vi "Recondense_mercury.vi"(5 "Recondense-Monitor in":T1 {"He3-Pot Heater %" format="%#_4g"; "He3-Pot Setpoint" format="%#_4g"; "Sorb Heater %" format="%#_4g"; "Sorb Setpoint" format="%#_4g"; "He3 Temp2" format="%#_4g"; "He3 Temp 1" format="%#_4g"; "1K Temp" format="%#_4g"; "Sorb Temp" format="%#_4g"}, 6 "TempErrorsIn":T7, 7 "Mercury Reference In H3 Temp2":T3, 8 "Mercury Reference In H3 Temp1":T3, 9 "Mercury Reference In 1K":T3, 10 "Mercury Reference In Sorb":T3) -> (0 "TempErrorsOut":T6, 2 "Mercury Reference out":T2, 3 "Recondense-Monitor out":T1 {"He3-Pot Heater %" format="%#_4g"; "He3-Pot Setpoint" format="%#_4g"; "Sorb Heater %" format="%#_4g"; "Sorb Setpoint" format="%#_4g"; "He3 Temp2" format="%#_4g"; "He3 Temp 1" format="%#_4g"; "1K Temp" format="%#_4g"; "Sorb Temp" format="%#_4g"})   [LabVIEW 2019]
uses:
  Equipment/Mercury iXX/Public/Controls/Mercury Reference.ctl
  Equipment/Mercury iXX/Public/Controls/Comms Transport Layer.ctl
  Equipment/Mercury iXX/Private/Controls/Query Dynamic Reference.ctl
  Monitor Communication/Brosowski/TempErrors_in.ctl
  Monitor Communication/Brosowski/TempErrors.ctl
  Monitor Communication/Brosowski/Mercury_Reference_out.ctl
  Monitor Communication/Brosowski/BorowskiMonitor.ctl
  Global/Global Variables/Data_Display_global.vi
  Equipment/Mercury iXX/Public/Libraries/Temperature.lvlib
  Equipment/Mercury iXX/Public/Libraries/Control Loop.lvlib
  Equipment/Mercury iXX/Mercury iXX.lvlib
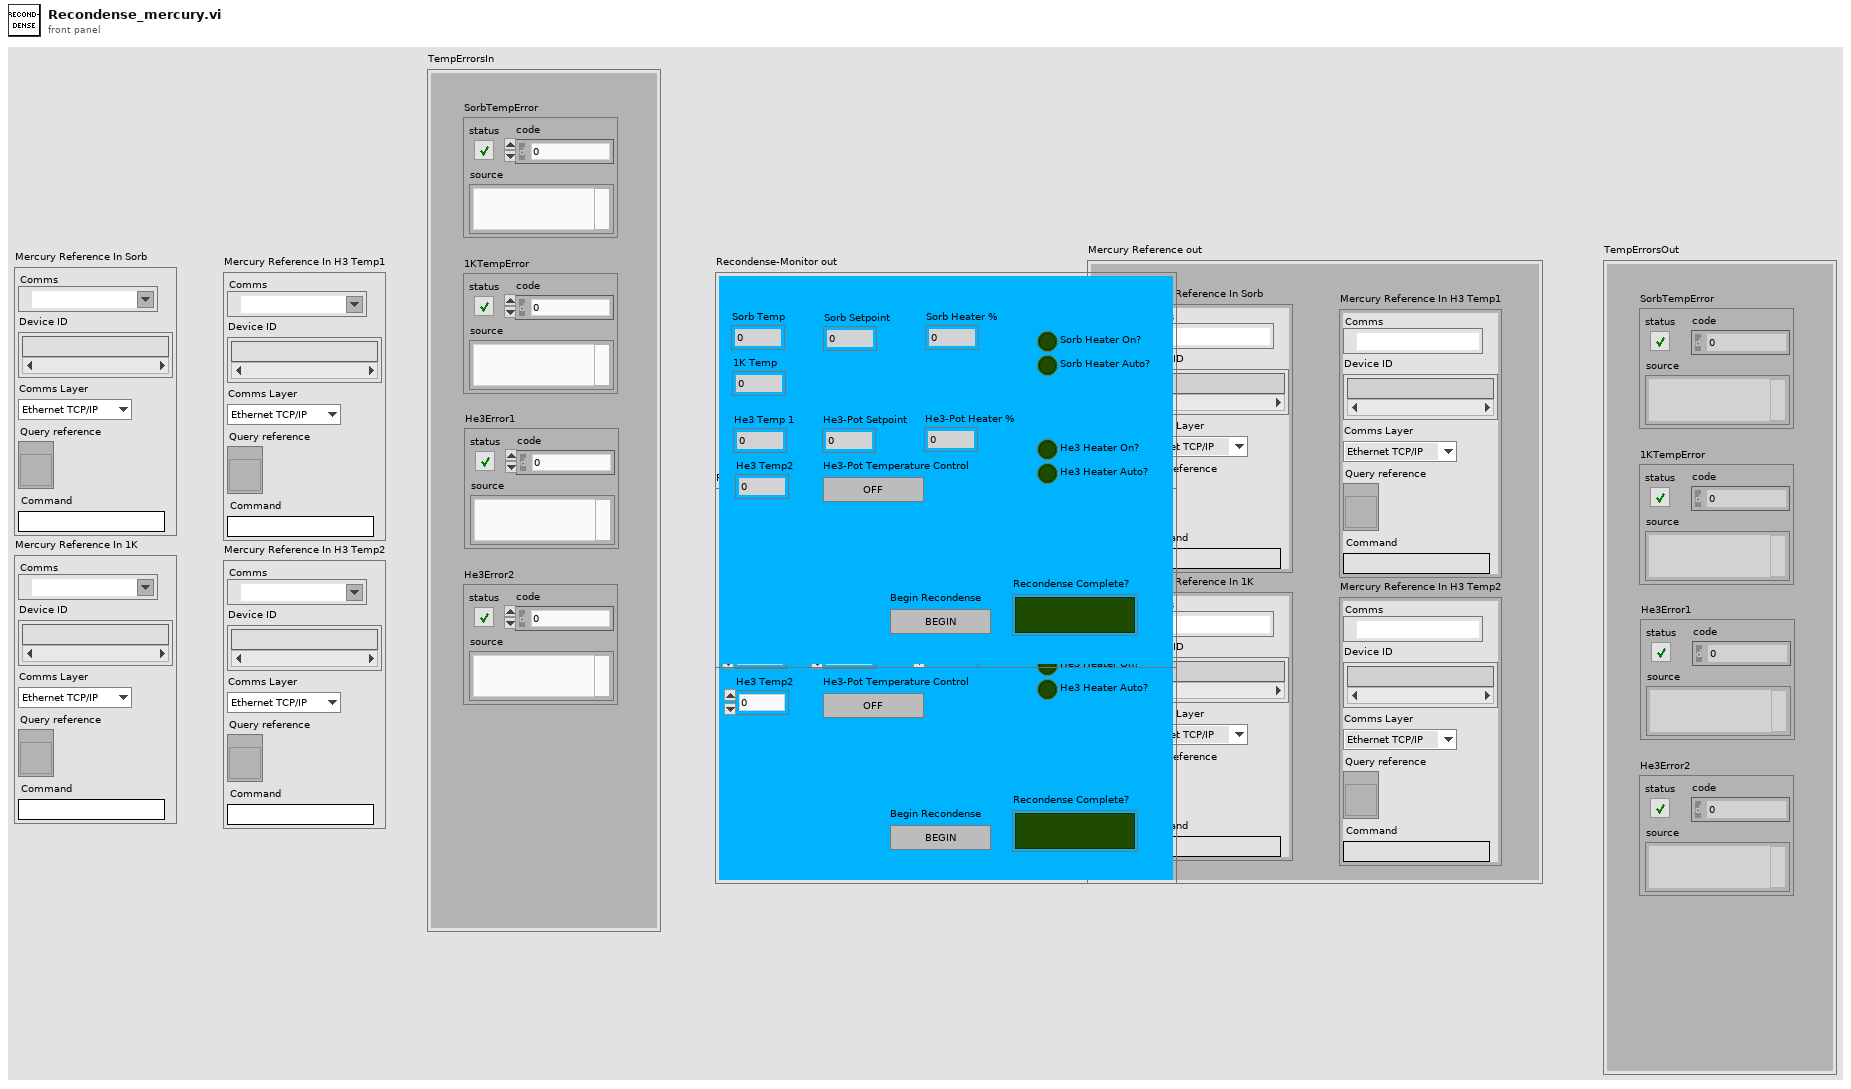
[diagram p1: front panel]
types:
  T1 = typedef "BorowskiMonitor.ctl" = cluster{"Sorb Temp":dbl, "1K Temp":dbl, "He3 Temp 1":dbl, "He3 Temp2":dbl, "Recondense Complete?":bool, "Sorb Heater Auto?":bool, "Sorb Heater On?":bool, "Sorb Setpoint":dbl, "Sorb Heater %":dbl, "Begin Recondense":bool, "He3-Pot Setpoint":dbl, "He3-Pot Heater %":dbl, "He3 Heater Auto?":bool, "He3 Heater On?":bool, "He3-Pot Temperature Control":bool}
  T2 = typedef "Mercury_Reference_out.ctl" = cluster{"Mercury Reference In Sorb":T3, "Mercury Reference In 1K":T3, "Mercury Reference In H3 Temp1":T3, "Mercury Reference In H3 Temp2":T3}
  T3 = typedef "Mercury iXX.lvlib/Mercury Reference.ctl" = cluster{"Comms":refnum<visa-resource-name>, "Device ID":string[], "Comms Layer":T4, "Command":string, "Query reference":T5}
  T4 = typedef "Mercury iXX.lvlib/Comms Transport Layer.ctl" = enum16{"Ethernet TCP/IP", "USB", "ISOBus - RS-232", "GPIB"}
  T5 = typedef "Mercury iXX.lvlib/Query Dynamic Reference.ctl" = refnum<vi>
  T6 = typedef "TempErrors.ctl" = cluster{"SorbTempError":errorcluster, "1KTempError":errorcluster, "He3Error1":errorcluster, "He3Error2":errorcluster}
  T7 = typedef "TempErrors_in.ctl" = cluster{"SorbTempError":errorcluster, "1KTempError":errorcluster, "He3Error1":errorcluster, "He3Error2":errorcluster}
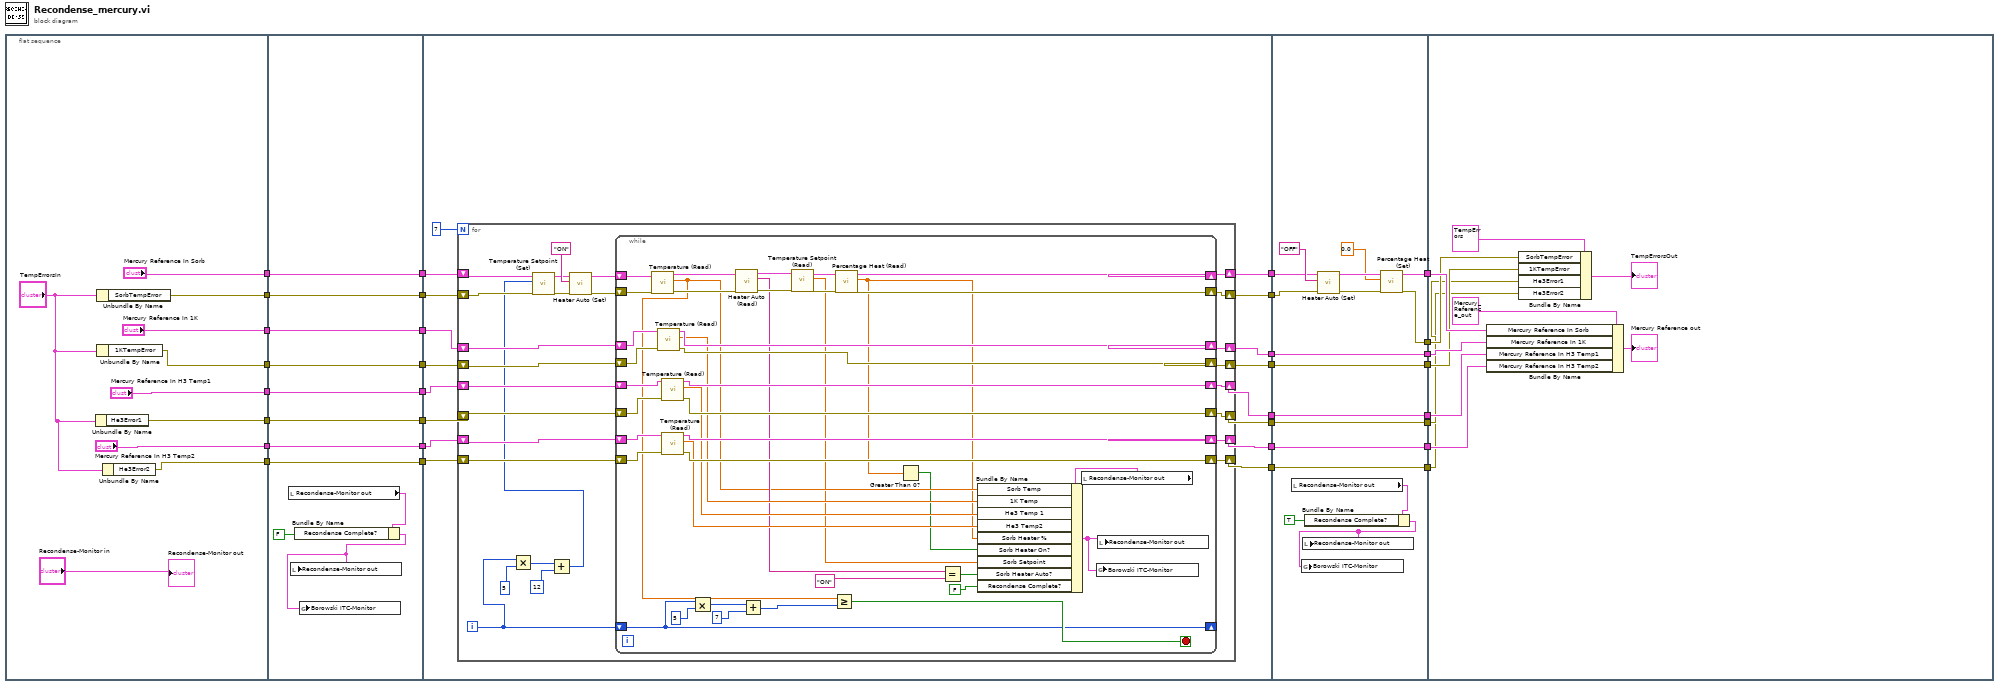
[diagram p0: block diagram]
diagram:
  n1 = flat-sequence {
    tunnel: ["Mercury Reference In Sorb"] -> w16
    tunnel: [w41] -> w14
    tunnel: ["Mercury Reference In 1K"] -> w12
    tunnel: [w39] -> w10
    tunnel: ["Mercury Reference In H3 Temp1"] -> w8
    tunnel: [w37] -> w6
    tunnel: ["Mercury Reference In H3 Temp2"] -> w4
    tunnel: [w34] -> w2
    tunnel: w16 -> [w53]
    tunnel: [w53] -> w15
    tunnel: w14 -> [w52]
    tunnel: [w52] -> w13
    tunnel: w12 -> [w51]
    tunnel: [w51] -> w11
    tunnel: w10 -> [w50]
    tunnel: [w50] -> w9
    tunnel: w8 -> [w49]
    tunnel: [w49] -> w7
    tunnel: w6 -> [w48]
    tunnel: [w48] -> w5
    tunnel: w4 -> [w47]
    tunnel: [w47] -> w3
    tunnel: w2 -> [w46]
    tunnel: [w46] -> w1
    tunnel: w15 -> [w69]
    tunnel: w13 -> [w68]
    tunnel: w11 -> [w67]
    tunnel: w9 -> [w66]
    tunnel: w7 -> [w65]
    tunnel: w5 -> [w64]
    tunnel: w3 -> [w63]
    tunnel: w1 -> [w62]
    tunnel: [w61] -> w32
    tunnel: [w60] -> w30
    tunnel: [w59] -> w28
    tunnel: [w58] -> w26
    tunnel: [w57] -> w24
    tunnel: [w56] -> w22
    tunnel: [w55] -> w20
    tunnel: [w54] -> w18
    tunnel: w32 -> [w144]
    tunnel: [w143] -> w31
    tunnel: w30 -> [w142]
    tunnel: [w141] -> w29
    tunnel: w28 -> [w154]
    tunnel: [w154] -> w27
    tunnel: w26 -> [w153]
    tunnel: [w153] -> w25
    tunnel: w24 -> [w152]
    tunnel: [w152] -> w23
    tunnel: w22 -> [w151]
    tunnel: [w151] -> w21
    tunnel: w20 -> [w150]
    tunnel: [w150] -> w19
    tunnel: w18 -> [w149]
    tunnel: [w149] -> w17
    tunnel: w31 -> [w166]
    tunnel: w29 -> [w164]
    tunnel: w27 -> [w160]
    tunnel: w25 -> [w159]
    tunnel: w23 -> [w156]
    tunnel: w21 -> [w158]
    tunnel: w19 -> [w155]
    tunnel: w17 -> [w157]
    frame #0 {
      n2 = Unbundle By Name("TempErrorsIn") -> ("He3Error1"=w37:errorcluster)
      n3 = Unbundle By Name("TempErrorsIn") -> ("SorbTempError"=w41:errorcluster)
      n4 = Unbundle By Name("TempErrorsIn") -> ("1KTempError"=w39:errorcluster)
      n5 = Unbundle By Name("TempErrorsIn") -> ("He3Error2"=w34:errorcluster)
      "Recondense-Monitor out" <- "Recondense-Monitor in"
    }
    frame #1 {
      n6 = local read "Recondense-Monitor out"() -> (w45:T1)
      n7 = Bundle By Name(cluster=w45, "Recondense Complete?"=FALSE) -> (w43:T1)
      n8 = local write "Recondense-Monitor out"(w43) -> ()
      n9 = global write "Data_Display_global.vi" "Borowski ITC-Monitor"(w43) -> ()
    }
    frame #2 {
      n10 = for {
        N: 7 -> [_]
        shift-right: [w85] -> w61
        shift-left: w69 -> [w77]
        shift-right: [w84] -> w60
        shift-left: w68 -> [w76]
        shift-right: [w83] -> w59
        shift-left: w67 -> [w90]
        shift-right: [w82] -> w54
        shift-left: w66 -> [w89]
        shift-right: [w81] -> w58
        shift-left: w65 -> [w88]
        shift-right: [w80] -> w57
        shift-left: w64 -> [w87]
        shift-right: [w79] -> w56
        shift-left: w63 -> [w86]
        shift-right: [w78] -> w55
        shift-left: w62 -> [w91]
        i -> [w72]
        n11 = Multiply(x=w72, y=5) -> (x*y=w74:i32)
        n12 = Add(x=w74, y=12) -> (x+y=w71:i32)
        n13 = call "Temperature Setpoint (Set).vi"("error in"=w76, "Temperature setpoint"=w71, "Mercury Reference In"=w77) -> ("error out"=w94:errorcluster, "Mercury Reference Out"=w95:T3)  [unwired: 5 in, 2 out]
        n14 = call "Heater Auto (Set).vi"("error in"=w94, "Heater Auto"="ON", "Mercury Reference In"=w95) -> ("error out"=w92:errorcluster, "Mercury Reference Out"=w93:T3)  [unwired: 5 in, 2 out]
        n15 = while {
          shift-right: [w114] -> w85
          shift-left: w93 -> [w137]
          shift-right: [w135] -> w83
          shift-left: w90 -> [w136]
          shift-right: [w133] -> w81
          shift-left: w88 -> [w134]
          shift-right: [w131] -> w79
          shift-left: w86 -> [w132]
          shift-right: [w113] -> w84
          shift-left: w92 -> [w124]
          shift-right: [w125] -> w82
          shift-left: w89 -> [w126]
          shift-right: [w127] -> w80
          shift-left: w87 -> [w128]
          shift-right: [w129] -> w78
          shift-left: w91 -> [w130]
          shift-right: [w108] -> _
          shift-left: w72 -> [w108]
          stop <- w109 stop-if-true
          n16 = call "Temperature (Read).vi"("error in"=w124, "Mercury Reference In"=w137) -> ("error out"=w111:errorcluster, "Temperature"=w110:dbl, "Mercury Reference Out"=w112:T3)  [unwired: 5 in, 2 out]
          n17 = call "Temperature (Read).vi"("error in"=w126, "Mercury Reference In"=w136) -> ("error out"=w125:errorcluster, "Temperature"=w121:dbl, "Mercury Reference Out"=w135:T3)  [unwired: 5 in, 2 out]
          n18 = call "Temperature (Read).vi"("error in"=w128, "Mercury Reference In"=w134) -> ("error out"=w127:errorcluster, "Temperature"=w120:dbl, "Mercury Reference Out"=w133:T3)  [unwired: 5 in, 2 out]
          n19 = call "Temperature (Read).vi"("error in"=w130, "Mercury Reference In"=w132) -> ("error out"=w129:errorcluster, "Temperature"=w122:dbl, "Mercury Reference Out"=w131:T3)  [unwired: 5 in, 2 out]
          n20 = Multiply(x=w108, y=5) -> (x*y=w106:i32)
          n21 = call "Heater Auto (Read).vi"("error in"=w111, "Mercury Reference In"=w112) -> ("error out"=w118:errorcluster, "Heater Auto"=w117:string, "Mercury Reference Out"=w119:T3)  [unwired: 6 in, 1 out]
          n22 = Add(x=w106, y=7) -> (x+y=w104:i32)
          n23 = call "Temperature Setpoint (Read).vi"("error in"=w118, "Mercury Reference In"=w119) -> ("error out"=w115:errorcluster, "Temperature Setpoint"=w102:dbl, "Mercury Reference Out"=w116:T3)  [unwired: 5 in, 2 out]
          n24 = Greater Or Equal?(x=w110, y=w104) -> (x >= y?=w109:bool)
          n25 = call "Percentage Heat (Read).vi"("error in"=w115, "Mercury Reference In"=w116) -> ("error out"=w113:errorcluster, "Percentage Heat"=w100:dbl, "Mercury Reference Out"=w114:T3)  [unwired: 5 in, 2 out]
          n26 = Greater Than 0?(x=w100) -> (x > 0?=w101:bool)
          n27 = Equal?(x=w117, y="ON") -> (x = y?=w99:bool)
          n28 = local read "Recondense-Monitor out"() -> (w123:T1)
          n29 = Bundle By Name(cluster=w123, "Sorb Temp"=w110, "1K Temp"=w121, "He3 Temp 1"=w120, "He3 Temp2"=w122, "Sorb Heater %"=w100, "Sorb Heater On?"=w101, "Sorb Setpoint"=w102, "Sorb Heater Auto?"=w99, "Recondense Complete?"=FALSE) -> (w97:T1)
          n30 = global write "Data_Display_global.vi" "Borowski ITC-Monitor"(w97) -> ()
          n31 = local write "Recondense-Monitor out"(w97) -> ()
        }
      }
    }
    frame #3 {
      n32 = local read "Recondense-Monitor out"() -> (w140:T1)
      n33 = Bundle By Name(cluster=w140, "Recondense Complete?"=TRUE) -> (w138:T1)
      n34 = global write "Data_Display_global.vi" "Borowski ITC-Monitor"(w138) -> ()
      n35 = local write "Recondense-Monitor out"(w138) -> ()
      n36 = call "Heater Auto (Set).vi"("error in"=w142, "Heater Auto"="OFF", "Mercury Reference In"=w144) -> ("error out"=w146:errorcluster, "Mercury Reference Out"=w147:T3)  [unwired: 5 in, 2 out]
      n37 = call "Percentage Heat (Set).vi"("error in"=w146, "Percentage Heat"=0.0, "Mercury Reference In"=w147) -> ("error out"=w141:errorcluster, "Mercury Reference Out"=w143:T3)  [unwired: 5 in, 2 out]
    }
    frame #4 {
      n38 = Bundle By Name(cluster=T2 {"Mercury Reference In Sorb"={"Comms"="", "Device ID"=[], "Comms Layer"=enum."Ethernet TCP/IP", "Command"="", "Query reference"=refnum}, "Mercury Reference In 1K"={"Comms"="", "Device ID"=[], "Comms Layer"=enum."Ethernet TCP/IP", "Command"="", "Query reference"=refnum}, "Mercury Reference In H3 Temp1"={"Comms"="", "Device ID"=[], "Comms Layer"=enum."Ethernet TCP/IP", "Command"="", "Query reference"=refnum}, "Mercury Reference In H3 Temp2"={"Comms"="", "Device ID"=[], "Comms Layer"=enum."Ethernet TCP/IP", "Command"="", "Query reference"=refnum}} ("Mercury Reference out"), "Mercury Reference In Sorb"=w166, "Mercury Reference In 1K"=w160, "Mercury Reference In H3 Temp1"=w159, "Mercury Reference In H3 Temp2"=w158) -> (→"Mercury Reference out":T2)
      n39 = Bundle By Name(cluster=T6 {"SorbTempError"={"status"=FALSE, "code"=0, "source"=""}, "1KTempError"={"status"=FALSE, "code"=0, "source"=""}, "He3Error1"={"status"=FALSE, "code"=0, "source"=""}, "He3Error2"={"status"=FALSE, "code"=0, "source"=""}} ("TempErrorsOut"), "SorbTempError"=w164, "1KTempError"=w157, "He3Error1"=w156, "He3Error2"=w155) -> (→"TempErrorsOut":T6)
    }
  }
